vi "FTW-Message-Request-Unknown.vi"(8 "error in":errorcluster, 11 "FTW Incoming Request":refnum<class "FTW-Message-HttpRequest.lvclass">) -> (0 "error out":errorcluster, 3 "FTW Incoming Request Out":refnum<class "FTW-Message-HttpRequest.lvclass">)   [LabVIEW 2015, in "FTW-Message-HttpRequest.lvclass"]
uses:
  FTW-Message-HttpRequest.lvclass
panel:
  # "Inputs"
  # "Outputs"
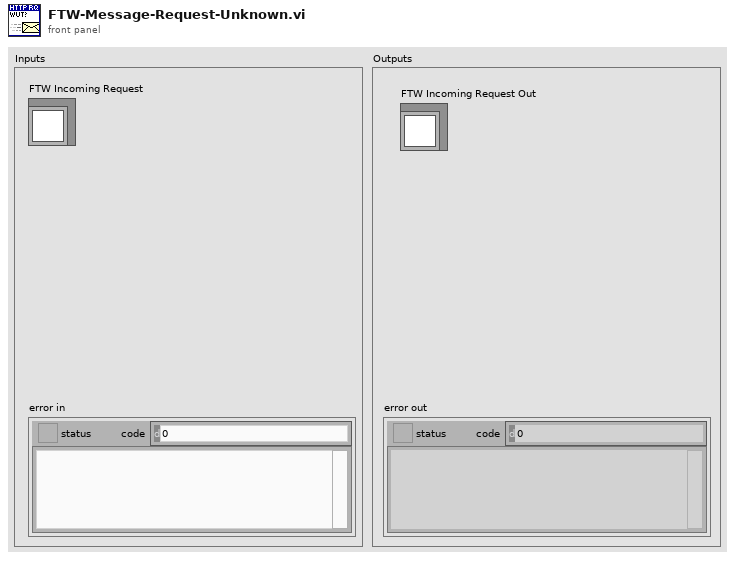
[diagram p1: front panel]
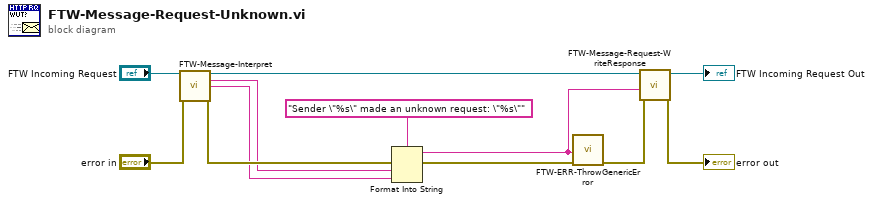
[diagram p0: block diagram]
diagram:
  n1 = call-dynamic "FTW-Message-Interpret.vi"("FTW Message"="FTW Incoming Request", "error in"="error in") -> ("FTW Message out"=w3:refnum<class "FTW-Message-HttpRequest.lvclass">, "Sender Identity"=w6:string, "Message Header"=w5:string, "error out"=w8:errorcluster)  [unwired: 9 in, 1 out]
  n2 = Format Into String(format string="Sender \"%s\" made an unknown request: \"%s\"", error in=w8, w6, w5) -> (resulting string=w1:string, error out=w9:errorcluster)  [unwired: 1 in]
  n3 = call "FTW-ERR-ThrowGenericError.vi"("Error Message"=w1, "error in"=w9) -> ("error out"=w7:errorcluster)  [unwired: 13 in]
  n4 = call "FTW-Message-Request-WriteResponse.vi"("error in"=w7, "Response Body"=w1, "FTW Incoming Request"=w3) -> ("error out"=→"error out":errorcluster, "FTW Incoming Request out"=→"FTW Incoming Request Out":refnum<class "FTW-Message-HttpRequest.lvclass">)  [unwired: 7 in]
